vi "7-Running Line.vi"() -> ()   [LabVIEW 2020]
panel:
  in  "milliseconds to wait(unit time)":u32=250
  in  "stop":bool
  out "Slide":string
  in  "n (letters per unit time)":i32=1
  in  "String":string="<User Name>"
  # "Since update of \"String\" control is triggered from an event case(value change),\nuser should change the string value in order to see the effect of sliding."
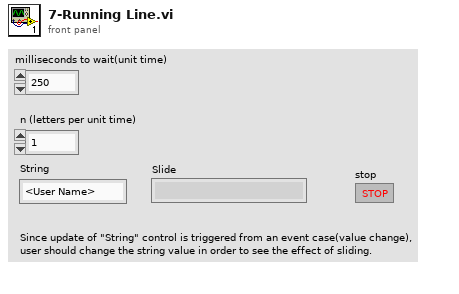
[diagram p1: front panel]
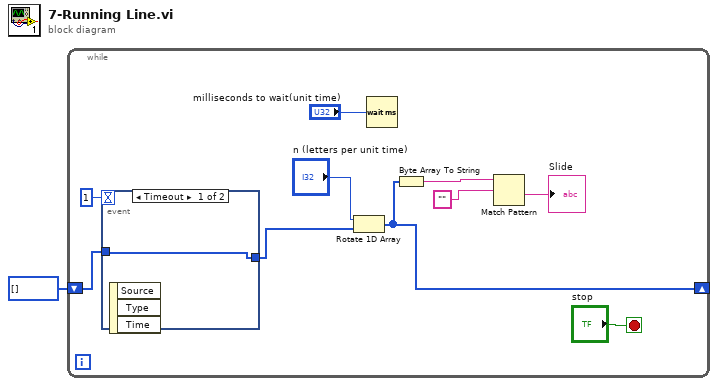
[diagram p0: block diagram]
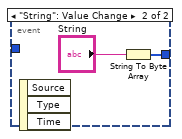
[diagram p2: hidden frame]
diagram:
  n1 = while {
    shift-right: [w5] -> _
    shift-left: u8[] [] -> [w2]
    stop <- "stop" stop-if-true
    n2 = event shown="[0] Timeout" {
      selector: _ -> [_ _]
      dyn-events: _ -> [_ _]
      timeout: 1 -> [_ _]
      tunnel: [w12 w13] -> w3
      tunnel: w2 -> [w12 _]
      event Timeout {
        n3 = event-data() -> ()  [unwired: 1 in, 3 out]
      }
      event "String": Value Change {
        n4 = event-data() -> ()  [unwired: 1 in, 3 out]
        n5 = String To Byte Array(string="String") -> (unsigned byte array=w13:u8[])
      }
    }
    n6 = Rotate 1D Array(1:w3, 2:"n (letters per unit time)") -> (0:w5:u8[])
    n7 = Wait (ms)(milliseconds to wait="milliseconds to wait(unit time)") -> ()  [unwired: 1 out]
    n8 = Byte Array To String(unsigned byte array=w5) -> (string=w10:string)
    n9 = Match Pattern(string=w10, regular expression="") -> (after substring=→"Slide":string)  [unwired: 1 in, 3 out]
  }
